vi "PDE Flexible Element.vi"() -> ()   [LabVIEW 2023]
doc: "This example demonstrates how to use the Partial Differential Equations VIs to define and solve a 2-dimensional Helmholtz equation on polygonal domain. The finite element method is used to solve the problem. One of the attractive features of this method is the flexibility in the choice of elements. In this example, the analytic solution varies dramatically in the center of the domain. Therefore, we specify dense grid, which results in small elements, in the center area of the domain. For this example, the flexible grid is able to find better solution than uniform grid.\n\nInstructions:\n1) Run the VI.\n2) Change the <b>Plot Style</b> to draw the solution with filled geometry or line segments.\n3) Change the <b>Sharpness</b> to see the difference when the variation of the solution becomes sharper or smoother in the center of the domain.\n4) Look at the block diagram for more information."
uses:
  <vilib>/gmath/pde.llb/Common/PDE_Plot Style.ctl
  <vilib>/gmath/pde.llb/Define 2D Helmholtz PDE (VIRef).vi
  <vilib>/gmath/pde.llb/Define 2D Helmholtz PDE BC (VIRef).vi
  <vilib>/gmath/pde.llb/Define 2D Helmholtz PDE Domain (Polygon).vi
  <vilib>/gmath/pde.llb/2D Helmholtz PDE Solver (Polygon Domain).vi
  <vilib>/gmath/pde.llb/2D Helmholtz PDE Rendering (Polygon Domain).vi
  <vilib>/gmath/NI_PDE.lvlib
panel:
  in  "Sharpness":dbl(slide)=0.01 scale=0.01..1.0 scale format="%#.2g"
  out "Solution on Uniform Grid":refnum<vi>(3d-picture)
  out "Analytic Solution":refnum<vi>(3d-picture)
  in  "Plot Style":T1=1 items=["Wireframe", "Polygons"]
  out "Solution on Flexible Grid":refnum<vi>(3d-picture)
  in  "Stop":bool
  # "Overview: This example demonstrates how to use the Partial Differential Equations VIs to define and solve a 2-dimensional Helmholtz equation on polygonal domain.\nRequirements: LabVIEW Full Development System\nInstructions: \n1. Run the VI.\n2. Change the Plot Style to draw the solution with filled geometry or line segments.\n3. Change the Sharpness to see the difference when the variation of the solution becomes sharper or smoother in the center of the domain.\n4. Click Stop to stop the VI."
  # "Sharper"
  # "Smoother"
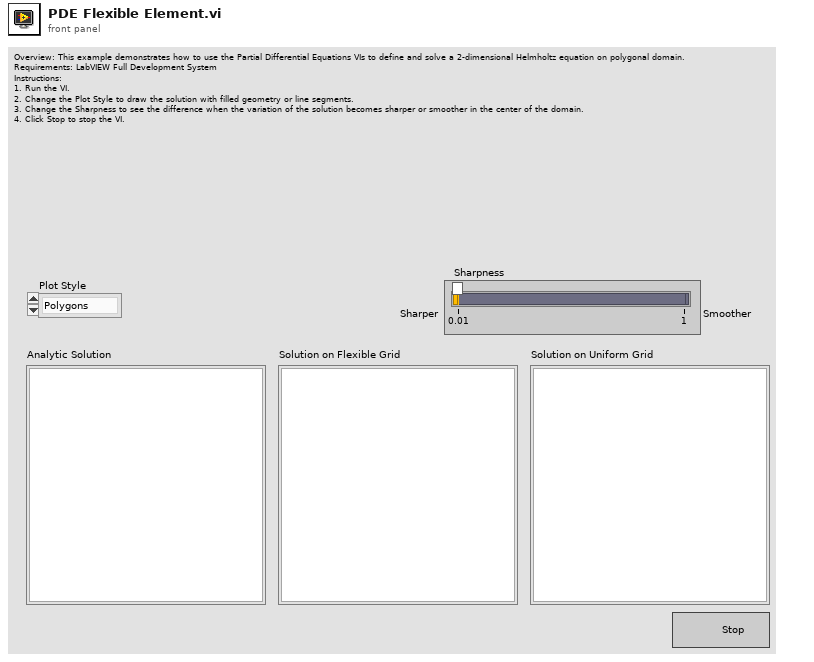
[diagram p1: front panel]
types:
  T1 = typedef "NI_PDE.lvlib/PDE_Plot Style.ctl" = i32
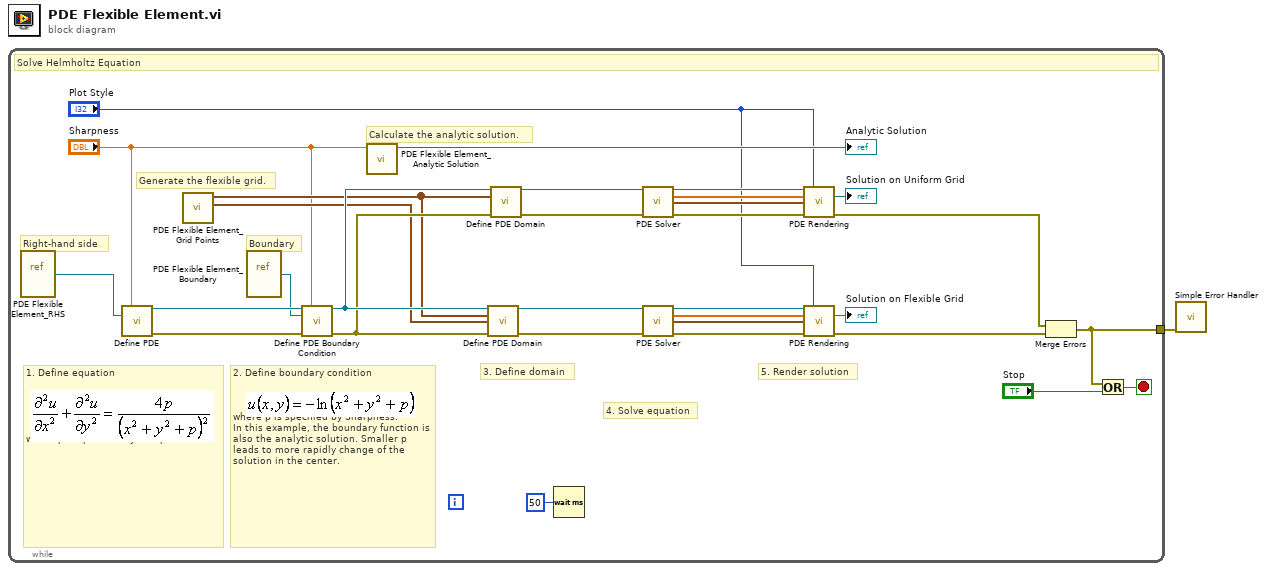
[diagram p0: block diagram]
diagram:
  n1 = while {
    tunnel: [w2] -> w1
    stop <- w4 stop-if-true
    # "Boundary"
    # "Right-hand side"
    # "Generate the flexible grid."
    # "Calculate the analytic solution."
    # "2. Define boundary condition\n\n\n\nwhere p is specified by Sharpness.\nIn this example, the boundary function is also the analytic solution. Smaller p leads to more rapidly change of the solution in the center."
    # "3. Define domain"
    # "1. Define equation\n\n\n\n\n\nwhere p is specified by Sharpness."
    # "4. Solve equation"
    # "5. Render solution"
    # "Solve Helmholtz Equation"
    n2 = vi-ref "PDE Flexible Element_RHS.vi"() -> (w21:refnum<vi>)
    n3 = call-poly <vilib>:"Define PDE.vi"("data"="Sharpness", "F(x, y)"=w21) -> ("PDE out"=w20:refnum<class "NI_PDE.lvclass">, "error out"=w19:errorcluster)  [unwired: 4 in, 8 out]
    n4 = call "PDE Flexible Element_Grid Points.vi"() -> ("Grid Points"=w10:cluster{"X":dbl, "Y":dbl}[], "Boundary Points"=w11:cluster{"X":dbl, "Y":dbl}[])  [unwired: 10 out]
    n5 = vi-ref "PDE Flexible Element_Boundary.vi"() -> (w18:refnum<vi>)
    n6 = call-poly <vilib>:"Define PDE Boundary Condition.vi"("PDE in"=w20, "data"="Sharpness", "Boundary Condition"=w18, "error in (no error)"=w19) -> ("PDE out"=w15:refnum<class "NI_PDE.lvclass">, "error out"=w14:errorcluster)  [unwired: 2 in, 8 out]
    n7 = call "PDE Flexible Element_Analytic Solution.vi"("data"="Sharpness") -> ("Analytic Sol"=→"Analytic Solution":refnum<vi>)  [unwired: 1 in, 9 out]
    n8 = call-poly <vilib>:"Define PDE Domain.vi"("PDE in"=w15, "Boundary Points"=w11, "Grid Points"=w10, "error in (no error)"=w14) -> ("PDE out"=w17:refnum<class "NI_PDE.lvclass">, "error out"=w16:errorcluster)  [unwired: 1 in, 9 out]
    n9 = call-poly <vilib>:"Define PDE Domain.vi"("PDE in"=w15, "Boundary Points"=w11, "error in (no error)"=w14) -> ("PDE out"=w12:refnum<class "NI_PDE.lvclass">, "error out"=w13:errorcluster)  [unwired: 2 in, 9 out]
    n10 = Wait (ms)(milliseconds to wait=u32 50) -> ()  [unwired: 1 out]
    n11 = call-poly <vilib>:"PDE Solver.vi"("PDE in"=w12, "error in (no error)"=w13) -> ("PDE out"=w27:refnum<class "NI_PDE.lvclass">, "U(x, y)"=w26:dbl[], "Grid Points"=w25:cluster{"X":dbl, "Y":dbl}[], "error out"=w28:errorcluster)  [unwired: 10 out]
    n12 = call-poly <vilib>:"PDE Solver.vi"("PDE in"=w17, "error in (no error)"=w16) -> ("PDE out"=w24:refnum<class "NI_PDE.lvclass">, "U(x, y)"=w23:dbl[], "Grid Points"=w22:cluster{"X":dbl, "Y":dbl}[], "error out"=w29:errorcluster)  [unwired: 10 out]
    n13 = call-poly <vilib>:"PDE Rendering.vi"("PDE in"=w27, "plot style"="Plot Style", "U(x, y)"=w26, "Grid Points"=w25, "error in (no error)"=w28) -> ("PDE Plot"=→"Solution on Uniform Grid":refnum<vi>, "error out"=w6:errorcluster)  [unwired: 9 out]
    n14 = call-poly <vilib>:"PDE Rendering.vi"("PDE in"=w24, "plot style"="Plot Style", "U(x, y)"=w23, "Grid Points"=w22, "error in (no error)"=w29) -> ("PDE Plot"=→"Solution on Flexible Grid":refnum<vi>, "error out"=w5:errorcluster)  [unwired: 9 out]
    n15 = Merge Errors(w6, w5) -> (w2:errorcluster)
    n16 = Or(x=w2, y="Stop") -> (x .or. y?=w4:bool)
  }
  n17 = call <vilib>:"Simple Error Handler.vi"("error in (no error)"=w1) -> ()  [unwired: 4 in, 5 out]
